vi "Run.vi"(8 "error in (no error)":errorcluster caption="entrée d'erreur (pas d'erreur)", 9 "y_score":string[][](array[string]), 10 "y_true":string[][](array[string]), 11 "Roc_Auc_Score.lvclass":refnum<class "Roc_Auc_Score.lvclass">) -> (0 "error out":errorcluster caption="sortie d'erreur", 2 "String Data":string, 3 "Roc_Auc_Score.lvclass":refnum<class "Roc_Auc_Score.lvclass">)   [LabVIEW 2020, in "Roc_Auc_Score.lvclass"]
doc: "Returns : \n\n- auc : float"
uses:
  Roc_Auc_Score.lvclass
  Roc_Auc_Score.lvclass/Roc_Auc_Score.ctl
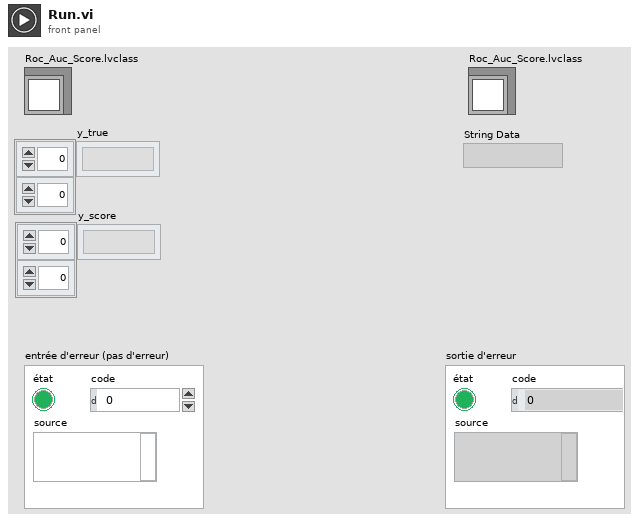
[diagram p1: front panel]
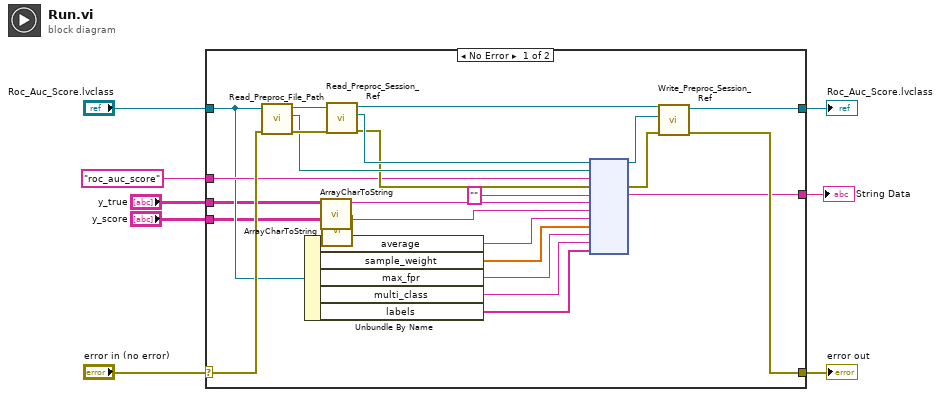
[diagram p0: block diagram]
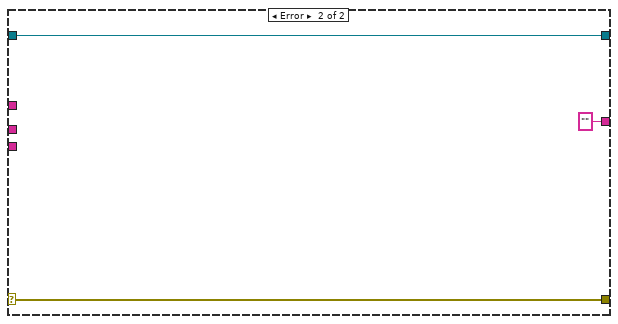
[diagram p2: hidden frame]
diagram:
  n1 = case shown="No Error" "error in (no error)" {
    selector: "error in (no error)" -> [w21 w35]
    tunnel: [w22 w35] -> w7
    tunnel: [w23 w34] -> w5
    tunnel: "Roc_Auc_Score.lvclass" -> [w18 w34]
    tunnel: "roc_auc_score" -> [w20 _]
    tunnel: [w19 ""] -> w4
    tunnel: "y_true" -> [w12 _]
    tunnel: "y_score" -> [w11 _]
    frame No Error {
      n2 = call-dynamic "Read_Preproc_File_Path.vi"("error in (no error)"=w21, "Python in"=w18) -> ("error out"=w31:errorcluster, "File_Path"=w30:path, "Python out"=w32:refnum<class "Roc_Auc_Score.lvclass">)  [unwired: 7 in]
      n3 = Unbundle By Name(w18) -> ("average"=w17:string, "sample_weight"=w16:dbl[], "max_fpr"=w15:string, "multi_class"=w14:string, "labels"=w13:string[])
      n4 = call "ArrayCharToString.vi"("TAB"=w12) -> ("Instruction"=w10:string)  [unwired: 10 in]
      n5 = call "ArrayCharToString.vi"("TAB"=w11) -> ("Instruction"=w9:string)  [unwired: 10 in]
      n6 = call-dynamic "Read_Preproc_Session_Ref.vi"("error in (no error)"=w31, "Python in"=w32) -> ("error out"=w28:errorcluster, "Session_ref"=w29:refnum<k35>, "Python out"=w27:refnum<class "Roc_Auc_Score.lvclass">)  [unwired: 7 in]
      n7 = node(w29, w30, w20, w28, "", w10, w9, w17, w16, w15, w14, w13) -> (w25:refnum<k35>, w26:errorcluster, w19:string)  [unwired: 7 in, 2 out]
      n8 = call-dynamic "Write_Preproc_Session_Ref.vi"("error in (no error)"=w26, "Session_ref"=w25, "Python in"=w27) -> ("error out"=w22:errorcluster, "Python out"=w23:refnum<class "Roc_Auc_Score.lvclass">)  [unwired: 7 in]
    }
    frame Error {
    }
  }
  "error out" <- w7
  "Roc_Auc_Score.lvclass" <- w5
  "String Data" <- w4
